vi "Init Device.vi"(7 "Layout Ref":refnum<vi>, 8 "error in (no error)":errorcluster, 10 "Chan# Array":i32[](array[numeric]), 11 "LTA-HS in":refnum<class "LTA-HS.lvclass">) -> (0 "error out":errorcluster, 3 "LTA-HS out":refnum<class "LTA-HS.lvclass">)   [LabVIEW 2013, in "LTA-HS.lvclass"]
doc: "Initialize the correct columns and their default appearance.\nUse the front panel to change default appearance of the device in the Add/Manage devices.\n\nOpen a specific device implementation for details."
uses:
  LTA-HS.lvclass
  TypeDefs/ColumnAppearCluster.ctl
  ColumnVIs/SingleValCol/SingleValCol.lvclass
  ColumnVIs/Column/Column.lvclass
panel:
  in  "Position Column Defaults":T1={"Column Name"="Frequency", "Width"=30, "Bkgd"=[16448250], "Text"=[0]}
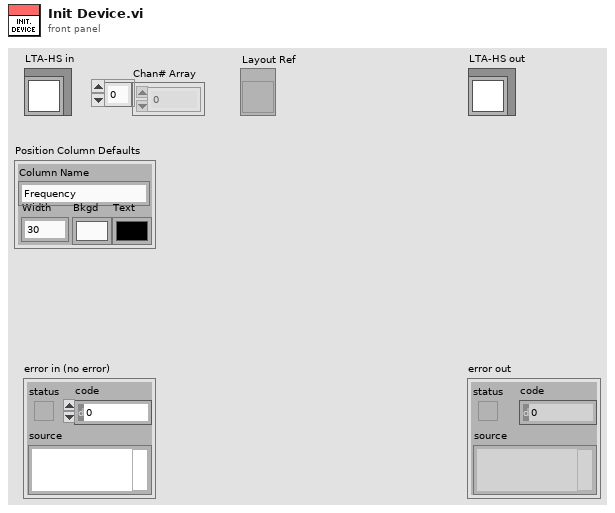
[diagram p1: front panel]
types:
  T1 = typedef "ColumnAppearCluster.ctl" = cluster{"Column Name":string, "Width":u32, "Bkgd":u32[], "Text":u32[]}
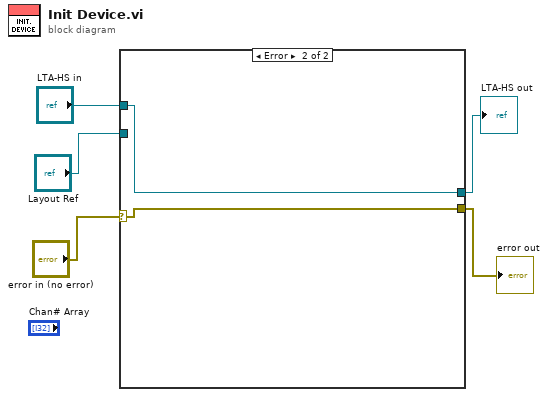
[diagram p0: block diagram]
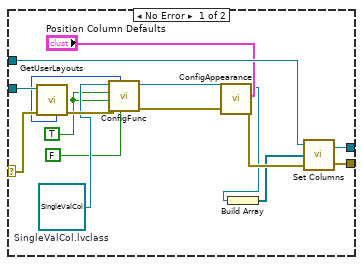
[diagram p2: hidden frame]
diagram:
  n1 = case shown="Error" "error in (no error)" {
    selector: "error in (no error)" -> [w21 w22]
    tunnel: "LTA-HS in" -> [w16 w23]
    tunnel: [w15 w23] -> w3
    tunnel: [w13 w22] -> w2
    tunnel: "Layout Ref" -> [w9 _]
    frame No Error {
      w11 = TRUE ("Disableable? (True)")
      w18 = refnum<class "SingleValCol.lvclass"> refnum  # SingleValCol.lvclass
      n2 = call "GetUserLayouts.vi"("error in (no error)"=w21, "Layout Ring Refnum"=w9) -> ("error out"=w20:errorcluster, "Num User Layouts"=w8:i32)  [unwired: 5 in, 3 out]
      n3 = call "ConfigFunc.vi"("isRampable? (True"=FALSE, "Num Layouts (ignored)"=w8, "error in (no error)"=w20, "isVariable? (True)"=w11, "Disableable? (True)"=w11, "Column in"=w18) -> ("error out"=w19:errorcluster, "Column out"=w17:refnum<class "SingleValCol.lvclass">)  [unwired: 4 in]
      n4 = call "ConfigAppearance.vi"("error in (no error)"=w19, "Column Appearance"="Position Column Defaults", "Column in"=w17) -> ("error out"=w14:errorcluster, "Column out"=w7:refnum<class "SingleValCol.lvclass">)  [unwired: 7 in]
      n5 = Build Array(w7) -> (w6:refnum<class "SingleValCol.lvclass">[])
      n6 = call-dynamic "Set Columns.vi"("error in (no error)"=w14, "Columns"=w6, "Device in"=w16) -> ("error out"=w13:errorcluster, "Device out"=w15:refnum<class "LTA-HS.lvclass">)  [unwired: 1 in]
    }
    frame Error {
    }
  }
  "error out" <- w2
  "LTA-HS out" <- w3
